vi "Find_Ch_data_start.vi"(3 "Start of read offset (chars.: 0)":i64, 4 "Approx No Of Columns":i32=1, 5 "Filename":path) -> (0 "Start of read offset output":i32, 1 "Titles and Data string":string, 2 "String before data":string)   [LabVIEW 2018]
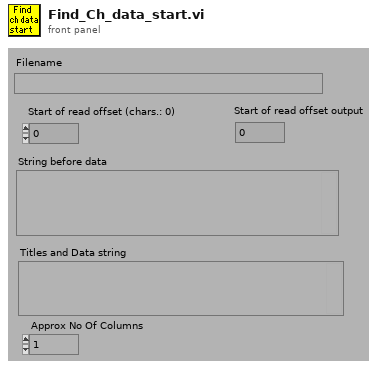
[diagram p1: front panel]
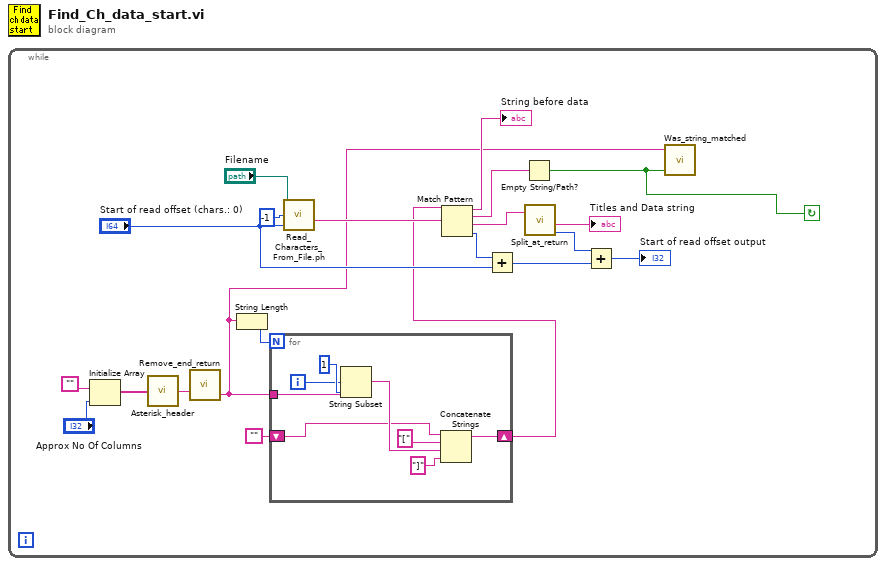
[diagram p0: block diagram]
diagram:
  n1 = while {
    stop <- w1 continue-if-true
    n2 = Initialize Array("", "Approx No Of Columns") -> (w19:string[])
    n3 = call "Asterisk_header.vi"("Channel names"=w19) -> ("Header string"=w6:string)
    n4 = call "Remove_end_return.vi"("Input string"=w6) -> ("Output string"=w2:string)
    n5 = String Length(string=w2) -> (length=w3:i32)
    n6 = for {
      N: w3 -> [_]
      tunnel: w2 -> [w25]
      shift-right: [w22] -> w4
      shift-left: "" -> [w23]
      i -> [w26]
      n7 = String Subset(string=w25, offset (0)=w26, length (rest)=1 ("length")) -> (substring=w24:string)
      n8 = Concatenate Strings(w23, "[", w24, "]" ("Substring")) -> (w22:string)
    }
    n9 = call "Read_Characters_From_File.ph.vi"("file path (dialog if empty)"="Filename", "number of characters (all:-1)"=-1, "start of read offset (chars.: 0)"="Start of read offset (chars.: 0)") -> ("character string"=w17:string)  [unwired: 6 out]
    n10 = Match Pattern(string=w17, regular expression=w4) -> (before substring=→"String before data":string, match substring=w10:string, after substring=w16:string, offset past match=w15:i32)  [unwired: 1 out]
    n11 = Add(x=w15, y="Start of read offset (chars.: 0)") -> (x+y=w12:i64)
    n12 = Empty String/Path?(string/path=w10) -> (empty?=w1:bool)
    n13 = call "Split_at_return.vi"("String"=w16) -> ("after substring"=→"Titles and Data string":string, "offset past match"=w13:i32)  [unwired: 1 in, 2 out]
    n14 = Add(x=w13, y=w12) -> (x+y=→"Start of read offset output":i64)
    n15 = call "Was_string_matched.vi"("Match Error"=w1, "Variable name"=w2) -> ()  [unwired: 1 in]
  }
